vi "init.vi"(8 "error in (no error)":errorcluster, 10 "WeatherData":refnum<class "WeatherData.lvclass">, 11 "CurrentConditionsDisplay in":refnum<class "StatisticsDisplay.lvclass">) -> (0 "error out":errorcluster, 3 "CurrentConditionsDisplay out":refnum<class "StatisticsDisplay.lvclass">)   [LabVIEW 2020, in "StatisticsDisplay.lvclass"]
uses:
  StatisticsDisplay.lvclass
  WeatherData/WeatherData.lvclass
  StatisticsData.ctl
  StatisticsDisplay.lvclass/StatisticsDisplay.ctl
  DisplayBase/DisplayBase.lvclass
panel:
  # "Connector Pane"
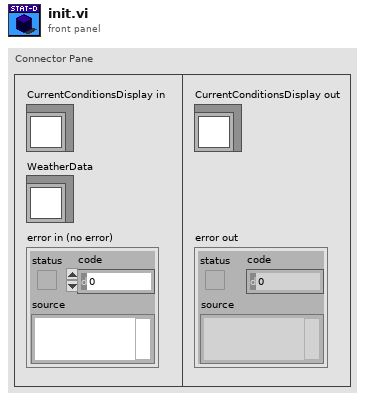
[diagram p1: front panel]
types:
  T1 = typedef "StatisticsDisplay.lvclass/StatisticsData.ctl" = cluster{"maxTemp":dbl, "minTemp":dbl, "TempSum":dbl, "nReadings":i32}
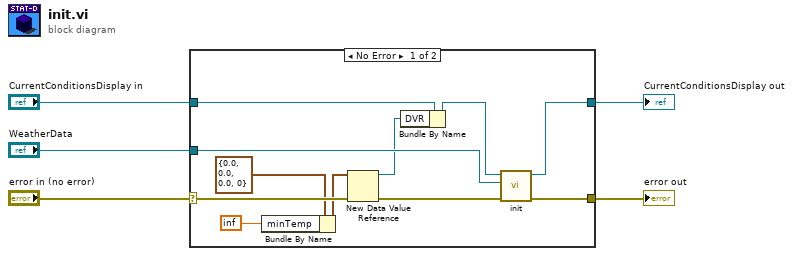
[diagram p0: block diagram]
diagram:
  n1 = case shown="No Error" "error in (no error)" {
    selector: "error in (no error)" -> [w12 w18]
    tunnel: [w16 w17] -> w5
    tunnel: "WeatherData" -> [w15 _]
    tunnel: "CurrentConditionsDisplay in" -> [w14 w17]
    tunnel: [w13 w18] -> w2
    frame No Error {
      n2 = Bundle By Name(cluster=T1 {"maxTemp"=0.0, "minTemp"=0.0, "TempSum"=0.0, "nReadings"=0} ("StatisticsData"), "minTemp"=inf) -> (w7:T1)
      n3 = New Data Value Reference(data value=w7, error in=w12) -> (data value reference=w8:refnum<data-value>, error out=w11:errorcluster)
      n4 = Bundle By Name(cluster=w14, "DVR"=w8) -> (w9:refnum<class "StatisticsDisplay.lvclass">)
      n5 = call-parent "init.vi"("error in (no error)"=w11, "WeatherData"=w15, "DisplayBase in"=w9) -> ("error out"=w13:errorcluster, "DisplayBase out"=w16:refnum<class "StatisticsDisplay.lvclass">)  [unwired: 7 in]
    }
    frame Error {
    }
  }
  "error out" <- w2
  "CurrentConditionsDisplay out" <- w5
